vi "Drive and Climb Logging Values.vi"() -> ()   [LabVIEW 2016]
panel:
  out "Right Drive Slave 2 Current":dbl
  out "Right Drive Slave 1 Current":dbl
  out "Right Drive Master Current":dbl
  out "Left Drive Slave 2 Current":dbl
  out "Left Drive Slave 1 Current":dbl
  out "Left Drive Master Current":dbl
  out "Current Drive Speed Gear":string="Low"
  out "Right Actual Velocity":dbl
  out "Right Drive Commanded Velocity":dbl
  out "Left Actual Velocity":dbl
  out "Left Drive Commanded Velocity":dbl
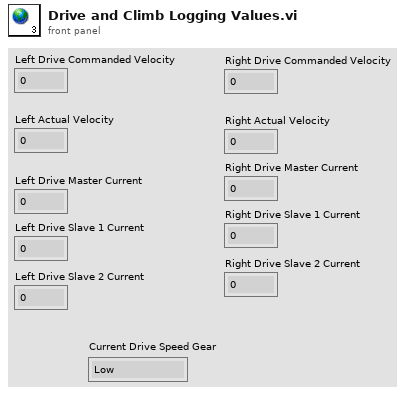
[diagram p1: front panel]
diagram:
